vi "Convert String to Enum - Window_Behaviour.vi"(8 "Error In":errorcluster, 11 "Window_Behaviour (string)":string) -> (0 "Error Out":errorcluster, 3 "Window_Behaviour (enum)":T1)   [LabVIEW 2016, in "Error Manager.lvlib" / "Settings.lvclass"]
doc: "This VI:\n1. Validates whether the input string represents a valid enum value\n2.1. If the above validation check passed, the VI converts the string value to the corresponding enum value\n2.2. If the validation check failed, the VI throws an error with an informative error message"
uses:
  Settings.lvclass
  <vilib>/Utility/Data Type/NI_Data Type.lvlib
  <vilib>/Utility/error.llb/whitespace.ctl
  Error Manager.lvlib
  Window_Behaviour (enum).ctl
panel:
  # "Development\nControls or indicators that are useful for development or testing, but which are not outputs of the VI."
  # "Input\nInputs to the VI"
  # "Output\nOutputs of the VI"
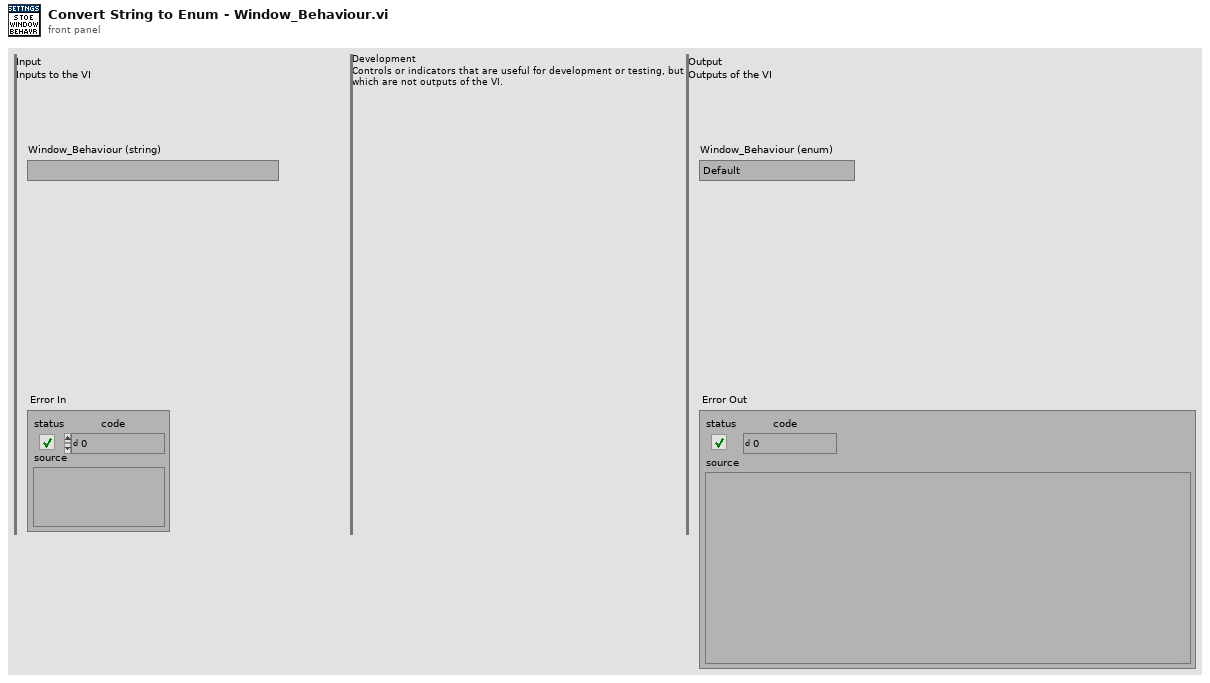
[diagram p1: front panel]
types:
  T1 = typedef "Error Manager.lvlib/Settings.lvclass/Window_Behaviour (enum).ctl" = enum16{"Default", "Floating", "Modal"}
  T2 = typedef "whitespace.ctl" = u16
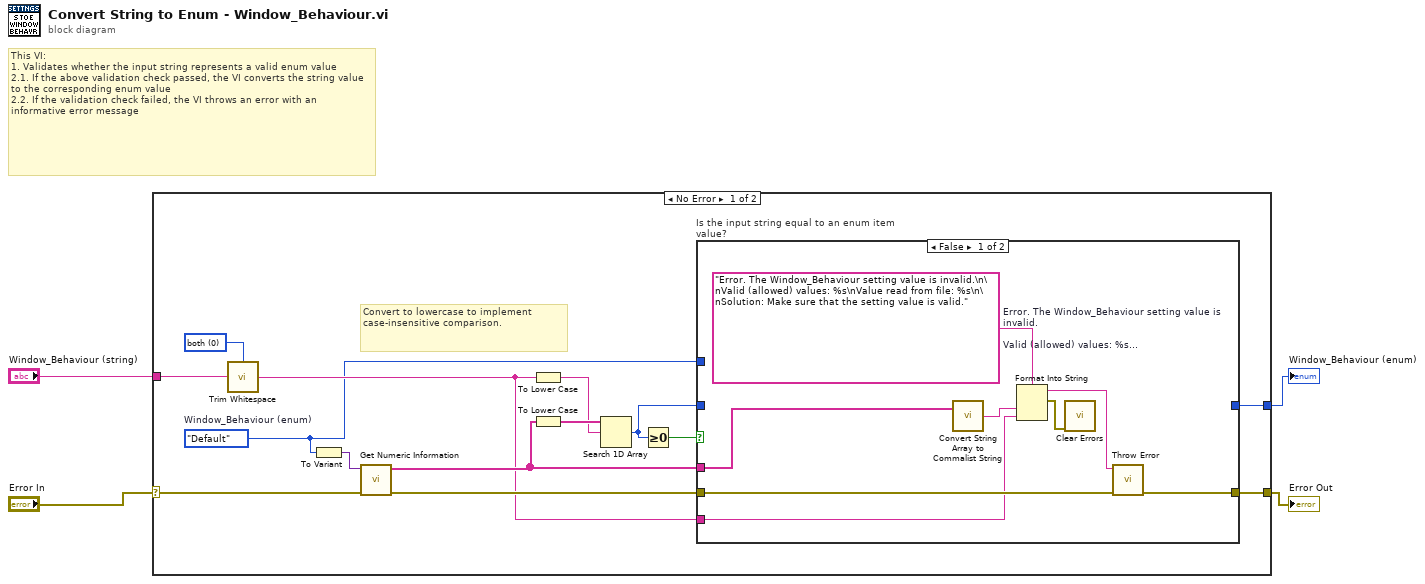
[diagram p0: block diagram]
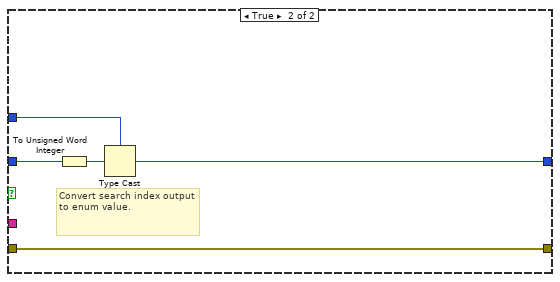
[diagram p2: hidden frame]
diagram:
  # "This VI:\n1. Validates whether the input string represents a valid enum value\n2.1. If the above validation check passed, the VI converts the string value to the corresponding enum value\n2.2. If the validation check failed, the VI throws an error with an informative error message"
  n1 = case shown="No Error" "Error In" {
    selector: "Error In" -> [w17 w32]
    tunnel: [w11 w32] -> w3
    tunnel: "Window_Behaviour (string)" -> [w14 _]
    tunnel: [w8 _] -> w1
    frame No Error {
      w5 = Window_Behaviour_(enum)."Default"  # Window_Behaviour (enum)
      w15 = T2 0 items=["both", "start of string", "end of string"] ("location (both)")
      # "Convert to lowercase to implement case-insensitive comparison."
      n2 = call <vilib>:"Trim Whitespace.vi"("string"=w14, "location (both)"=w15) -> ("trimmed string"=w6:string)
      n3 = To Variant(anything=w5) -> (Variant=w18:variant)
      n4 = call <vilib>:"Get Numeric Information.vi"("error in (no error)"=w17, "variant"=w18) -> ("error out"=w16:errorcluster, "enum names"=w7:string[])  [unwired: 6 in, 2 out]
      n5 = To Lower Case(string=w6) -> (all lower case string=w12:string)
      n6 = To Lower Case(string=w7) -> (all lower case string=w13:string[])
      n7 = Search 1D Array(1D array=w13, element=w12) -> (index of element=w9:i32)  [unwired: 1 in]
      n8 = Greater Or Equal To 0?(x=w9) -> (x >= 0?=w10:bool)
      n9 = case "Is the input string equal to an enum item value?" shown="False" w10 {
        tunnel: w16 -> [w26 w31]
        tunnel: [w25 w31] -> w11
        tunnel: w9 -> [_ w30]
        tunnel: w5 -> [_ w28]
        tunnel: [_ w27] -> w8
        tunnel: w7 -> [w21 _]
        tunnel: w6 -> [w20 _]
        frame False {
          w23 = "Error. The Window_Behaviour setting value is invalid.\n\nValid (allowed) values: %s\nValue read from file: %s\n\nSolution: Make sure that the setting value is valid."  # Error. The Window_Behaviour setting value is invalid.  Valid (allowed) values: %s Value read from file: %s  Solution: Make sure that the setting value is valid.
          n10 = call "Convert String Array to Commalist String.vi"("String Array"=w21) -> ("Commalist string"=w22:string)  [unwired: 1 in]
          n11 = Format Into String(format string=w23, w22, w20) -> (resulting string=w19:string, error out=w24:errorcluster)  [unwired: 2 in]
          n12 = call <vilib>:"Clear Errors.vi"("error in (no error)"=w24) -> ()  [unwired: 5 in, 2 out]
          n13 = call "Throw Error.vi"("error in"=w26, "Error Message"=w19) -> ("error out"=w25:errorcluster)  [unwired: 9 in]
        }
        frame True {
          # "Convert search index output to enum value."
          n14 = To Unsigned Word Integer(number=w30) -> (unsigned 16bit integer=w29:u16)
          n15 = Type Cast(type=w28, x=w29) -> (*(type *) &x=w27:T1)
        }
      }
    }
    frame Error {
    }
  }
  "Error Out" <- w3
  "Window_Behaviour (enum)" <- w1
